vi "UTIL_Calibrate.vi"() -> ()   [LabVIEW 2024]
panel:
  out "Cal_High_Oil_Level":string
  out "Cal_High_Laser_Reading":string
  out "Cal_Low_Laser_Reading":string
  out "Cal_Low_Oil_Level":string
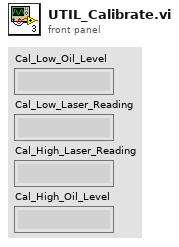
[diagram p1: front panel]
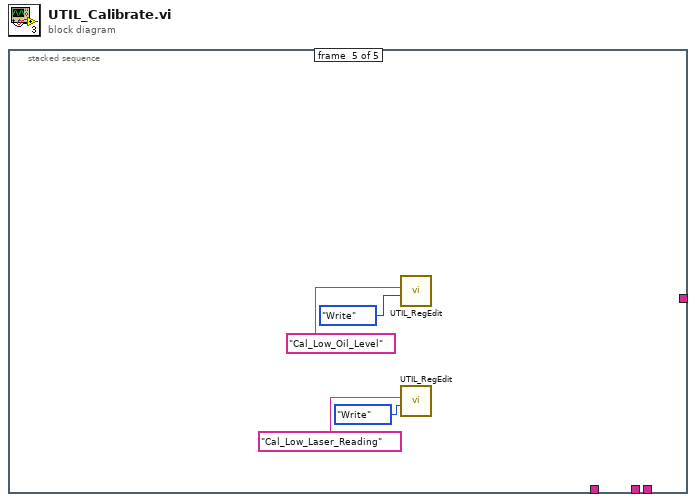
[diagram p0: block diagram]
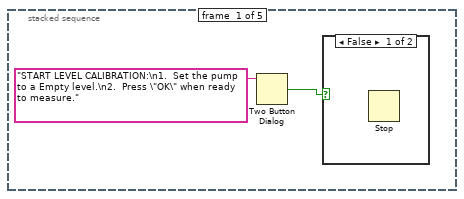
[diagram p2: hidden frame]
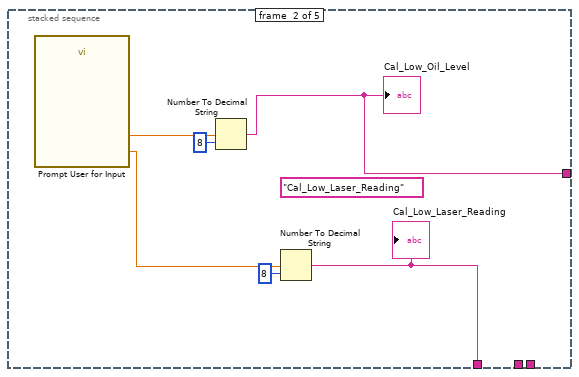
[diagram p4: hidden frame]
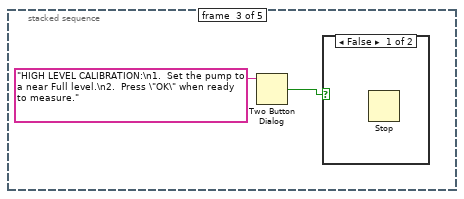
[diagram p5: hidden frame]
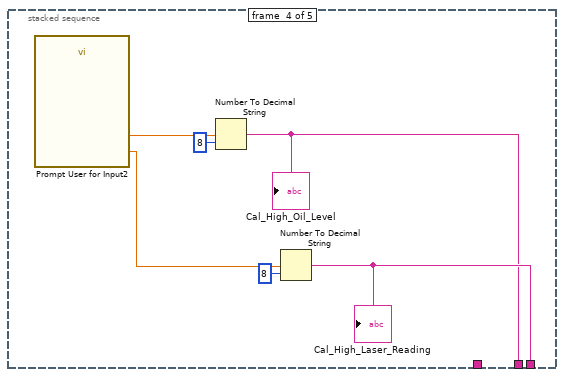
[diagram p7: hidden frame]
diagram:
  n1 = stacked-sequence {
    tunnel: [_ w4 _ _ _] -> _
    tunnel: [_ _ _ w12 _] -> _
    tunnel: [_ _ _ w11 _] -> _
    tunnel: [_ w3 _ _ _] -> _
    frame #0 {
      n2 = Two Button Dialog(message="START LEVEL CALIBRATION:\n1.  Set the pump to a Empty level.\n2.  Press \"OK\" when ready to measure.") -> (T button?=w1:bool)  [unwired: 2 in]
      n3 = case shown="False" w1 {
        frame False {
          n4 = Stop() -> ()  [unwired: 1 in]
        }
        frame True {
        }
      }
    }
    frame #1 {
      (unwired) "Cal_Low_Laser_Reading"
      n5 = call "Prompt User for Input"() -> ("Low Laser Reading"=w5:dbl, "Low Measurement"=w8:dbl)  [unwired: 16 in, 2 out]
      n6 = Number To Decimal String(number=w8, width (-)=i16 8) -> (decimal integer string=w3:string)
      "Cal_Low_Oil_Level" <- w3
      n7 = Number To Decimal String(number=w5, width (-)=i16 8) -> (decimal integer string=w4:string)
      "Cal_Low_Laser_Reading" <- w4
    }
    frame #2 {
      n8 = Two Button Dialog(message="HIGH LEVEL CALIBRATION:\n1.  Set the pump to a near Full level.\n2.  Press \"OK\" when ready to measure.") -> (T button?=w9:bool)  [unwired: 2 in]
      n9 = case shown="False" w9 {
        frame False {
          n10 = Stop() -> ()  [unwired: 1 in]
        }
        frame True {
        }
      }
    }
    frame #3 {
      n11 = call "Prompt User for Input2"() -> ("Low Laser Reading"=w13:dbl, "Low Measurement"=w16:dbl)  [unwired: 16 in, 2 out]
      n12 = Number To Decimal String(number=w16, width (-)=i16 8) -> (decimal integer string=w11:string)
      "Cal_High_Oil_Level" <- w11
      n13 = Number To Decimal String(number=w13, width (-)=i16 8) -> (decimal integer string=w12:string)
      "Cal_High_Laser_Reading" <- w12
    }
    frame #4 {
      n14 = call "UTIL_RegEdit.vi"("Mode"=enum16{"Write", "Read", "Delete"}."Write", "String Name"="Cal_Low_Oil_Level") -> ()  [unwired: 8 in, 2 out]
      n15 = call "UTIL_RegEdit.vi"("Mode"=enum16{"Write", "Read", "Delete"}."Write", "String Name"="Cal_Low_Laser_Reading") -> ()  [unwired: 8 in, 2 out]
    }
  }
